vi "controlAQuadBOutResolution.vi"(7 "Set":bool, 8 "error in":errorcluster, 9 "ABoutRes in":i32, 10 "axis in":u8, 11 "connection ID":refnum<k5>) -> (0 "error out":errorcluster, 1 "ABoutRes out":i32, 2 "axis out":u8, 3 "connection ID":refnum<k5>)   [LabVIEW 2016]
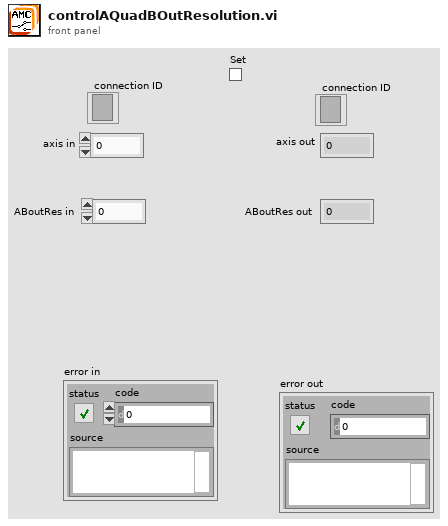
[diagram p1: front panel]
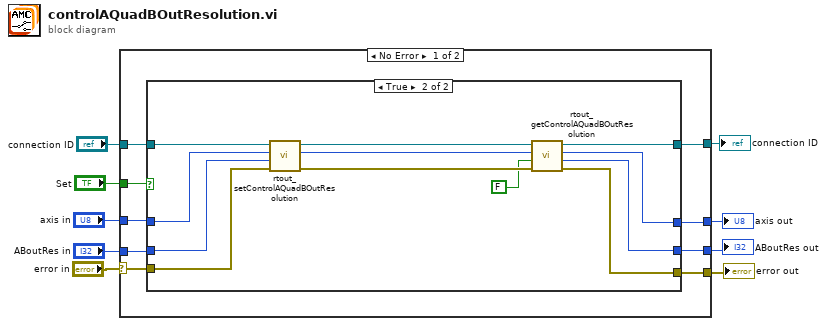
[diagram p0: block diagram]
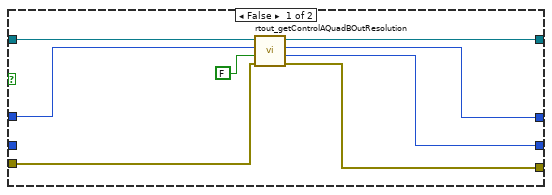
[diagram p2: hidden frame]
diagram:
  n1 = case shown="No Error" "error in" {
    selector: "error in" -> [w10 w41]
    tunnel: "axis in" -> [w16 w40]
    tunnel: [w11 w41] -> w8
    tunnel: [w13 w40] -> w7
    tunnel: "Set" -> [w17 _]
    tunnel: [w14 w39] -> w5
    tunnel: "connection ID" -> [w18 w39]
    tunnel: "ABoutRes in" -> [w15 w42]
    tunnel: [w12 w42] -> w2
    frame No Error {
      n2 = case shown="True" w17 {
        tunnel: [w25 w33] -> w14
        tunnel: w18 -> [w26 w38]
        tunnel: w16 -> [w22 w36]
        tunnel: [w21 w29] -> w13
        tunnel: [w19 w30] -> w12
        tunnel: [w23 w31] -> w11
        tunnel: w15 -> [_ w35]
        tunnel: w10 -> [w24 w37]
        frame False {
          n3 = call "rtout_getControlAQuadBOutResolution.vi"("error in"=w24, "tempvalue"=FALSE, "axis"=w22, "connection ID"=w26) -> ("error out"=w23:errorcluster, "resolution"=w19:i32, "axis_out"=w21:i32, "connection ID"=w25:refnum<k5>)  [unwired: 4 in]
        }
        frame True {
          n4 = call "rtout_setControlAQuadBOutResolution.vi"("error in"=w37, "resolution"=w35, "axis"=w36, "connection ID"=w38) -> ("error out"=w32:errorcluster, "axis_out"=w28:i32, "connection ID"=w34:refnum<k5>)  [unwired: 5 in]
          n5 = call "rtout_getControlAQuadBOutResolution.vi"("error in"=w32, "tempvalue"=FALSE, "axis"=w28, "connection ID"=w34) -> ("error out"=w31:errorcluster, "resolution"=w30:i32, "axis_out"=w29:i32, "connection ID"=w33:refnum<k5>)  [unwired: 4 in]
        }
      }
    }
    frame Error {
    }
  }
  "error out" <- w8
  "axis out" <- w7
  "connection ID" <- w5
  "ABoutRes out" <- w2
